vi "Request Data JSON.vi"(8 "error in (no error)":errorcluster, 11 "CreateProfile in":refnum<class "CreateProfile.lvclass">) -> (0 "error out":errorcluster, 2 "Request Data JSON":string, 3 "CreateProfile out":refnum<class "CreateProfile.lvclass">)   [LabVIEW 2022 SP3, in "obs-websocket-lv.lvlib" / "CreateProfile.lvclass"]
uses:
  CreateProfile.lvclass
  CreateProfile.lvclass/CreateProfile.ctl
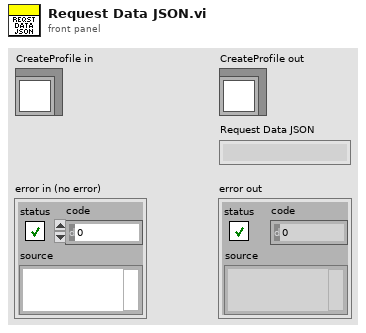
[diagram p1: front panel]
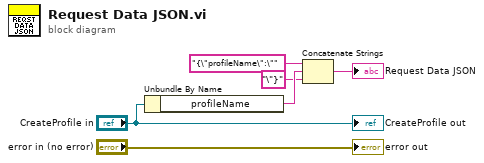
[diagram p0: block diagram]
diagram:
  n1 = Unbundle By Name("CreateProfile in") -> ("profileName"=w4:string)
  n2 = Concatenate Strings("{\"profileName\":\"" ("string"), w4, "\"}" ("string")) -> (→"Request Data JSON":string)
  "error out" <- "error in (no error)"
  "CreateProfile out" <- "CreateProfile in"
